vi "manual_test_random.vi"(5 "change_in_event":refnum<user-event>, 7 "waitgroup":T1, 8 "error in (no error)":errorcluster, 11 "data":variant) -> (0 "error out":errorcluster)   [LabVIEW 2015, in "example_01.lvlib"]
uses:
  example_01.lvlib
  <userlib>/antonio-alexander/lv-waitgroup/public/_controls/api_waitgroup.ctl
  lv-recipe-machine/public/_controls/change.ctl
  _controls/step_data.ctl
  _controls/manual_actions.ctl
  lv-recipe-machine/lv-recipe-machine.lvlib
  <userlib>/antonio-alexander/lv-waitgroup/lv-waitgroup.lvlib
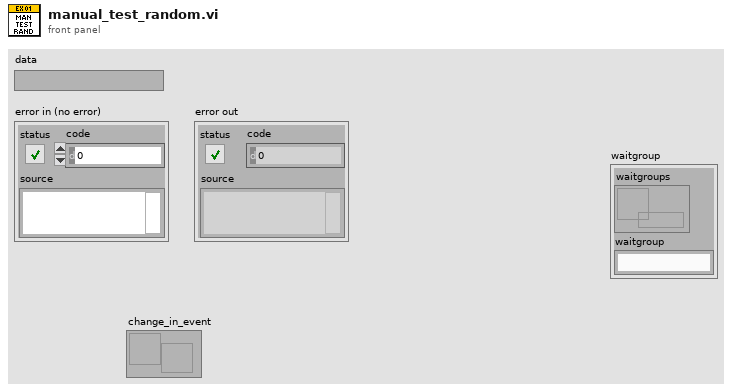
[diagram p1: front panel]
types:
  T1 = typedef "lv-waitgroup.lvlib/api_waitgroup.ctl" = cluster{"waitgroups":refnum<data-value>, "waitgroup":string}
  T2 = typedef "example_01.lvlib/manual_actions.ctl" = enum16{"<manual_action>", "manual_test_random", "manual_test_comparison", "manual_test_wait", "<null>"}
  T3 = typedef "example_01.lvlib/step_data.ctl" = cluster{"data":variant, "step":string}
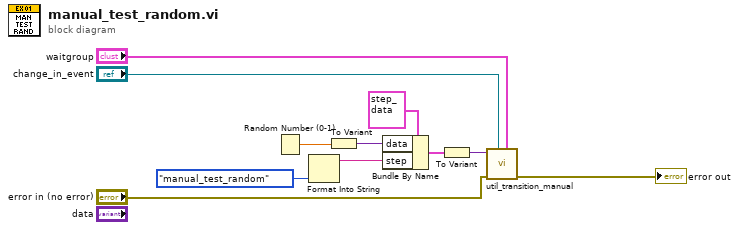
[diagram p0: block diagram]
diagram:
  n1 = Random Number (0-1)() -> (number: 0 to 1=w8:dbl)
  n2 = Format Into String(manual_actions."manual_test_random" ("manual_action")) -> (resulting string=w6:string)  [unwired: 3 in, 1 out]
  n3 = To Variant(anything=w8) -> (Variant=w5:variant)
  n4 = Bundle By Name(cluster=T3 {"data"=variant, "step"=""}, "data"=w5, "step"=w6) -> (w9:T3)
  n5 = To Variant(anything=w9) -> (Variant=w4:variant)
  n6 = call "util_transition_manual.vi"("api_waitgroup"="waitgroup", "change_in_event"="change_in_event", "error in (no error)"="error in (no error)", "data"=w4) -> ("error out"=→"error out":errorcluster)  [unwired: 7 in]
